vi "parse start line.vi"(8 "error in":errorcluster, 10 "initial scan location":u32, 11 "String":string) -> (0 "error out":errorcluster, 1 "URL":string, 2 "HTTP method":T2, 3 "remaining string":string, 4 "HTTP protocol version":T1, 5 "offset past scan":u32)   [LabVIEW 2019, in "WebSocket Server Toolkit.lvlib"]
uses:
  WebSocket Server Toolkit.lvlib
  types/HTTP Request Method.ctl
  types/HTTP Protocol Version.ctl
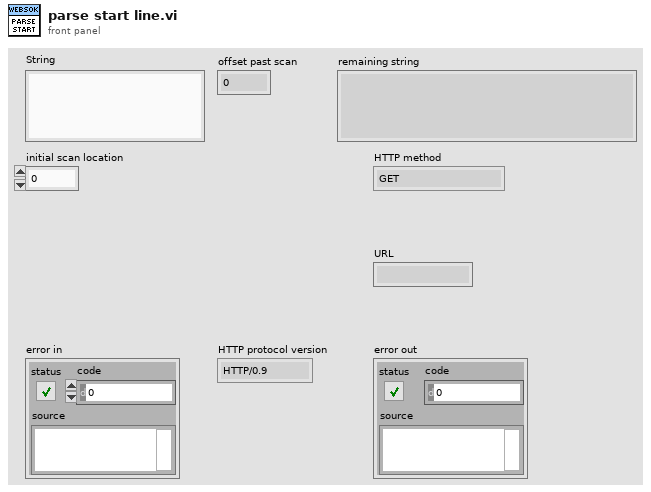
[diagram p1: front panel]
types:
  T1 = typedef "WebSocket Server Toolkit.lvlib/HTTP Protocol Version.ctl" = enum16{"HTTP/0.9", "HTTP/1.0", "HTTP/1.1", "HTTP/2.0", "HTTP/3.0"}
  T2 = typedef "WebSocket Server Toolkit.lvlib/HTTP Request Method.ctl" = enum16{"GET", "HEAD", "POST", "PUT", "DELETE", "CONNECT", "OPTIONS", "TRACE", "PATCH"}
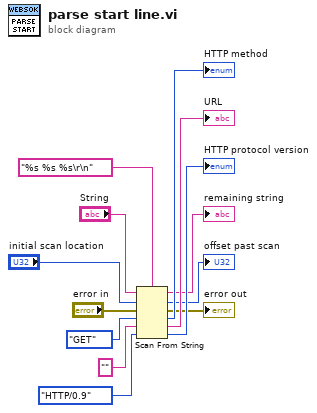
[diagram p0: block diagram]
diagram:
  n1 = Scan From String(format string="%s %s %s\r\n", input string="String", initial scan location="initial scan location", error in="error in", default 1=HTTP_Request_Method."GET" ("HTTP Method"), default 2="" ("default value 2"), default 3=HTTP_Protocol_Version."HTTP/0.9" ("HTTP version")) -> (remaining string=→"remaining string":string, offset past scan=→"offset past scan":u32, error out=→"error out":errorcluster, output 1=→"HTTP method":T2, output 2=→"URL":string, output 3=→"HTTP protocol version":T1)
